vi "Get Strings from Enum TD__ogtk.vi"(8 "error in (no error)":errorcluster, 10 "Type Descriptor":i16[](array[numeric])) -> (0 "error out":errorcluster, 1 "enum name":string, 2 "enum strings":string[](array[string]))   [LabVIEW 2019]
doc: "Returns Enum Strings array, String Value and Enum Name from an Enum Type Descriptor."
panel:
  # "[OpenG VI Tags] ***Do Not Remove***"
  # "Get Strings from Enum TD.vi\n\nReturns Enum Strings array, String Value and Enum Name from an Enum Type Descriptor.\n\nPlease visit http://www.OpenG.org to learn about the\nOpen Source LabVIEW software movement.\n\nNOTICE -- YOU MUST LEAVE THIS NOTICE IN PLACE.  PER THE TERMS OF THE LICENSE BELOW, YOU MAY SUBLICENSE THIS SOFTWARE \nIN ANY WAY THAT DOES NOT CONFLICT WITH THIS LICENSE.\n\n### BSD License (http://www.opensource.org/licenses/bsd-license.php) Begin ###\n \nCopyright (c) 2002, Jean-Pierre Drolet <drolet_jp@hotmail.com>\nCopyright (c) 2002-2006, Jim Kring <jim@jimkring.com>\n\nAll rights reserved.\n\nRedistribution and use in source and binary forms, with or without modification, are permitted provided that the following conditions are met:\n\n    * Redistributions of source code must retain the above copyright notice, this list of conditions and the following disclaimer.\n    * Redistributions in binary form must reproduce the above copyright notice, this list of conditions and the following disclaimer in the \n       documentation and/or other materials provided with the distribution.\n    * Neither the name of SciWare, James Kring, Inc., nor the names of its contributors may be used to endorse or promote products derived \n       from this software without specific prior written permission.\n\nTHIS SOFTWARE IS PROVIDED BY THE COPYRIGHT HOLDERS AND CONTRIBUTORS \"AS IS\" AND ANY EXPRESS OR IMPLIED WARRANTIES, \nINCLUDING, BUT NOT LIMITED TO, THE IMPLIED WARRANTIES OF MERCHANTABILITY AND FITNESS FOR A PARTICULAR PURPOSE ARE \nDISCLAIMED. IN NO EVENT SHALL THE COPYRIGHT OWNER OR CONTRIBUTORS BE LIABLE FOR ANY DIRECT, INDIRECT, INCIDENTAL,\n SPECIAL, EXEMPLARY, OR CONSEQUENTIAL DAMAGES (INCLUDING, BUT NOT LIMITED TO, PROCUREMENT OF SUBSTITUTE GOODS OR \nSERVICES; LOSS OF USE, DATA, OR PROFITS; OR BUSINESS INTERRUPTION) HOWEVER CAUSED AND ON ANY THEORY OF LIABILITY, \nWHETHER IN CONTRACT, STRICT LIABILITY, OR TORT (INCLUDING NEGLIGENCE OR OTHERWISE) ARISING IN ANY WAY OUT OF THE USE \nOF THIS SOFTWARE, EVEN IF ADVISED OF THE POSSIBILITY OF SUCH DAMAGE.\n\n### BSD License End ###"
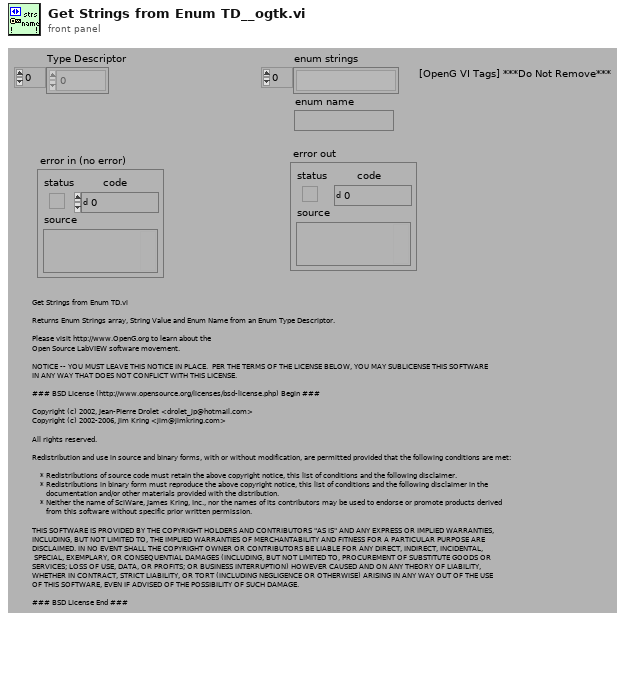
[diagram p1: front panel]
types:
  T1 = typedef "Type Descriptor Header__ogtk.ctl" = cluster{"length":u16, "private":u8, "type":T2, "# elements":u16}
  T2 = typedef "Type Descriptor Enumeration__ogtk.ctl" = enum8{"<Null>", "I8", "I16", "I32", "I64", "U8", "U16", "U32", "U64", "SGL", "DBL", "EXT", "CSG", "CDB", "CXT", "0x0F", "0x10", "0x11", "0x12", "0x13", "0x14", "Enum U8", "Enum U16", "Enum U32", "Enum U64", "SGL PQ", "DBL PQ", "EXT PQ", "CSG PQ", "CDB PQ", "CXT PQ", "0x1F", "0x20", "Boolean", "0x22", "0x23", "0x24", "0x25", "0x26", "0x27", "0x28", "0x29", "0x2A", "0x2B", "0x2C", "0x2D", "0x2E", "0x2F", "String", "0x31", "Path", "Pict", "0x34", "0x35", "0x36", "DAQ", "0x38", "0x39", "0x3A", "0x3B", "0x3C", "0x3D", "0x3E", "0x3F", "Array", "0x41", "0x42", "0x43", "0x44", "0x45", "0x46", "0x47", "0x48", "0x49", "0x4A", "0x4B", "0x4C", "0x4D", "0x4E", "0x4F", "Cluster", "0x51", "0x52", "Variant", "Waveform", "0x55", "0x56", "0x57", "0x58", "0x59", "0x5A", "0x5B", "0x5C", "0x5D", "0x5E", "Fixed Point", "0x60", "0x61", "0x62", "0x63", "0x64", "0x65", "0x66", "0x67", "0x68", "0x69", "0x6A", "0x6B", "0x6C", "0x6D", "0x6E", "0x6F", "Refnum", "0x71", "0x72", "Set Collection", "Map Collection"}
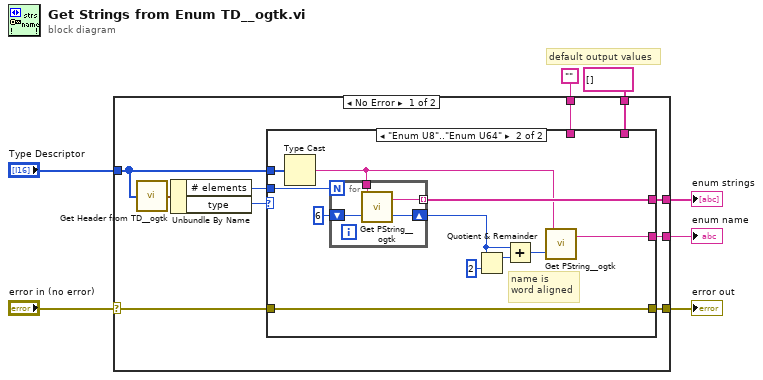
[diagram p0: block diagram]
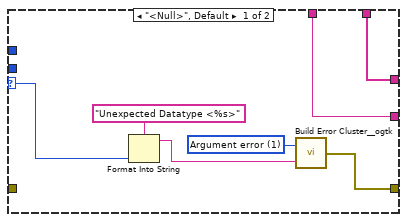
[diagram p2: hidden frame]
diagram:
  # "default output values"
  n1 = case shown="No Error" "error in (no error)" {
    selector: "error in (no error)" -> [w8 w40]
    tunnel: [w9 w40] -> w7
    tunnel: "Type Descriptor" -> [w15 _]
    tunnel: [w14 w42] -> w5
    tunnel: [w13 w41] -> w4
    tunnel: string[] [] -> [w11 w42]
    tunnel: "" ("PString") -> [w10 w41]
    frame No Error {
      n2 = call "Get Header from TD__ogtk.vi"("Type Descriptor"=w15) -> ("Type Descriptor Header"=w16:T1)
      n3 = Unbundle By Name(w16) -> ("# elements"=w17:u16, "type"=w12:T2)
      n4 = case shown="\"Enum U8\"..\"Enum U64\"" w12 {
        selector: w12 -> [w19 _]
        tunnel: w17 -> [_ w35]
        tunnel: w15 -> [_ w34]
        tunnel: [w24 w33] -> w14
        tunnel: [w23 w32] -> w13
        tunnel: w11 -> [w24 _]
        tunnel: w10 -> [w23 _]
        tunnel: [w18 w25] -> w9
        tunnel: w8 -> [_ w25]
        frame "<Null>", Default {
          w22 = 1 items=["No error", "Argument error", "Memory is full", "Out of zone", "End of file", "File already open", "Generic file I/O error", "File not found", "File permission error", "Disk is full", "Duplicate path", "Too many files open", "System feature not enabled", "Resource file not found", "Cannot add resource", "Resource not found", "Image not found", "Image memory error", "Pen does not exist", "Config type invalid", "Config token not found", "Config parse error", "Config memory error", "Bad external code format", "Bad external code offset", "External code not present", "Null window", "Destroy window error", "Null menu", "Print aborted", "Bad print record", "Print driver error", "Windows error during printing", "Memory error during printing", "Print dialog error", "Generic print error", "Invalid device refnum", "Device not found", "Device parameter error", "Device unit error", "Cannot open device", "Device call aborted", "Generic error", "Cancelled by user", "Object ID too low", "Object ID too high", "Object not in heap", "Unknown heap", "Unknown object (invalid DefProc)", "Unknown object (DefProc not in table)", "Message out of range", "Invalid (null) method", "Unknown message", "Manager call not supported", "Bad address", "Network operation in progress", "Network operation timed out", "Connection is busy", "Network attribute not supported", "Network error", "Address in use", "System out of memory", "Connection aborted", "Connection refused", "Not connected", "Already connected", "Connection closed", "Initialization error (interapplication manager)", "Bad occurrence", "Wait on unbound occurrence handler", "Occurrence queue overflow", "Datalog type conflict", "Unused", "Unrecognized type (interapplication manager)", "Memory corrupt", "Failed to make temporary DLL", "Old CIN version", "Drag socket not found", "Failed to load drop-object", "Failed to register OLE object", "Failed to release OLE object", "Format specifier type mismatch", "Unknown format specifier", "Too few format specifiers", "Too many format specifiers", "Scan failed", "Newer CIN version", "Error converting to variant", "Runtime menu error", "Password tampered", "Variant attribute not found", "Incompatible variant data type", "Event data is not available", "Event Store is not present", "Occurrence is not found", "Event Queue is not created", "Event info is not available", "Refnum passed is NULL", "Error retrieving Class GUID", "Error retrieving CoClass GUID", "Error retrieving TypeLib GUID.", "Bad built application magic bytes.", "Specific driver is different from the specific driver associated with the Logical Name.", "There is no session opened to the class driver.", "Max Error", "MAX - Error with config objects", "MAX - Error loading configuration", "MAX - Group not supported"]
          n5 = Format Into String(format string="Unexpected Datatype <%s>" ("Format String"), w19) -> (resulting string=w20:string)  [unwired: 2 in, 1 out]
          n6 = call "Build Error Cluster__ogtk.vi"("String to Prepend to source (\"\")"=w20, "code"=w22) -> ("error out"=w18:errorcluster)
        }
        frame "Enum U8".."Enum U64" {
          # "name is\nword aligned"
          n7 = Type Cast(x=w34) -> (*(type *) &x=w30:string)  [unwired: 1 in]
          n8 = for {
            N: w35 -> [_]
            tunnel: w30 -> [w36]
            shift-right: [w37] -> w29
            shift-left: 6 -> [w38]
            tunnel: [w39] -> w33 mode=indexing
            n9 = call "Get PString__ogtk.vi"("offset (0)"=w38, "String"=w36) -> ("offset past PString"=w37:i32, "PString"=w39:string)
          }
          n10 = Quotient & Remainder(x=w29, y=2) -> (x-y*floor(x/y)=w28:i32)  [unwired: 1 out]
          n11 = Add(x=w29, y=w28) -> (x+y=w31:i32)
          n12 = call "Get PString__ogtk.vi"("offset (0)"=w31, "String"=w30) -> ("PString"=w32:string)  [unwired: 1 out]
        }
      }
    }
    frame Error {
    }
  }
  "error out" <- w7
  "enum strings" <- w5
  "enum name" <- w4
